vi "Disconnect.vi"(8 "error in (no error)":errorcluster, 11 "Protocol in":refnum<class "Protocol.lvclass">) -> (0 "error out":errorcluster, 3 "Protocol out":refnum<class "Protocol.lvclass">)   [LabVIEW 2020, in "CSM-FileSync.lvlib" / "Protocol.lvclass"]
uses:
  Protocol.lvclass
  Protocol.lvclass/Protocol.ctl
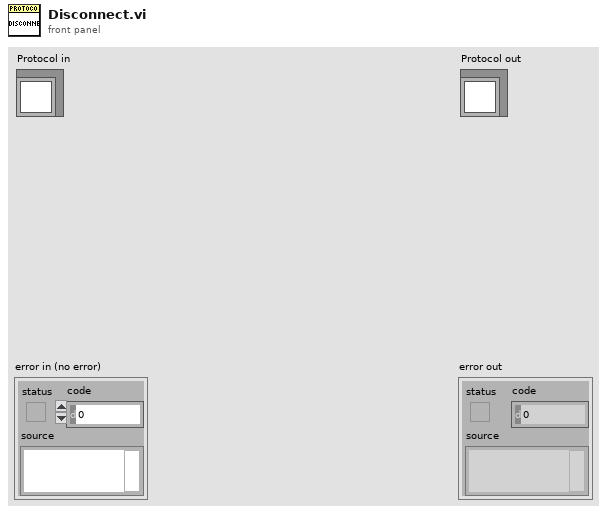
[diagram p1: front panel]
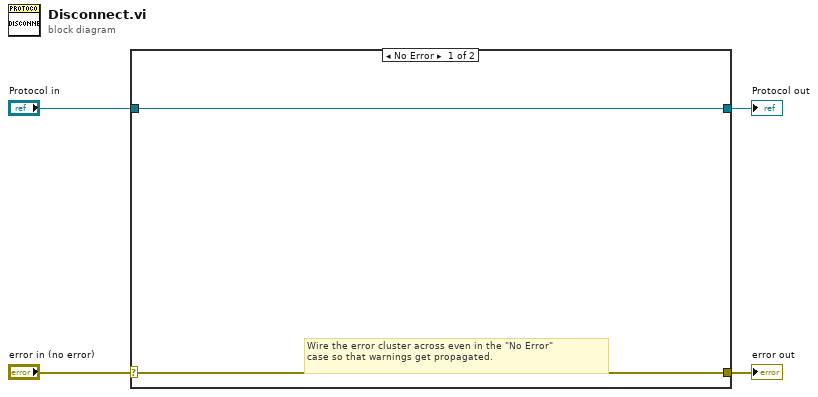
[diagram p0: block diagram]
diagram:
  n1 = case shown="No Error" "error in (no error)" {
    selector: "error in (no error)" -> [w5 w8]
    tunnel: [w5 w8] -> w3
    tunnel: [w6 w7] -> w1
    tunnel: "Protocol in" -> [w6 w7]
    frame No Error {
      # "Wire the error cluster across even in the \"No Error\"\ncase so that warnings get propagated."
    }
    frame Error {
    }
  }
  "error out" <- w3
  "Protocol out" <- w1
